vi "Defragment.vi"(11 "Path":path) -> (0 "error out":errorcluster)   [LabVIEW 2019, in "TDMS.lvlib" / "TDMS.lvclass"]
uses:
  TDMS.lvclass
panel:
  in  "Cancel Button":bool
  out "Processing Report Please Wait":dbl(slide) scale=0.0..100.0
  # "%"
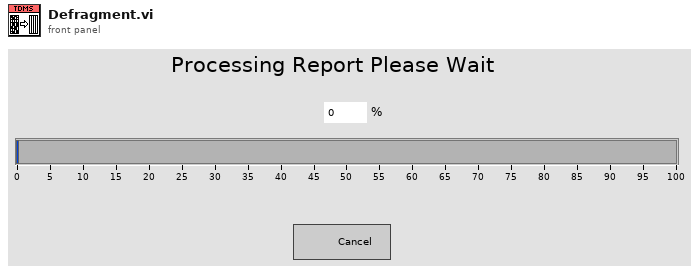
[diagram p1: front panel]
types:
  T1 = enum32{"Invalid", "Standard", "Closed", "Hidden", "Minimized", "Maximized"}
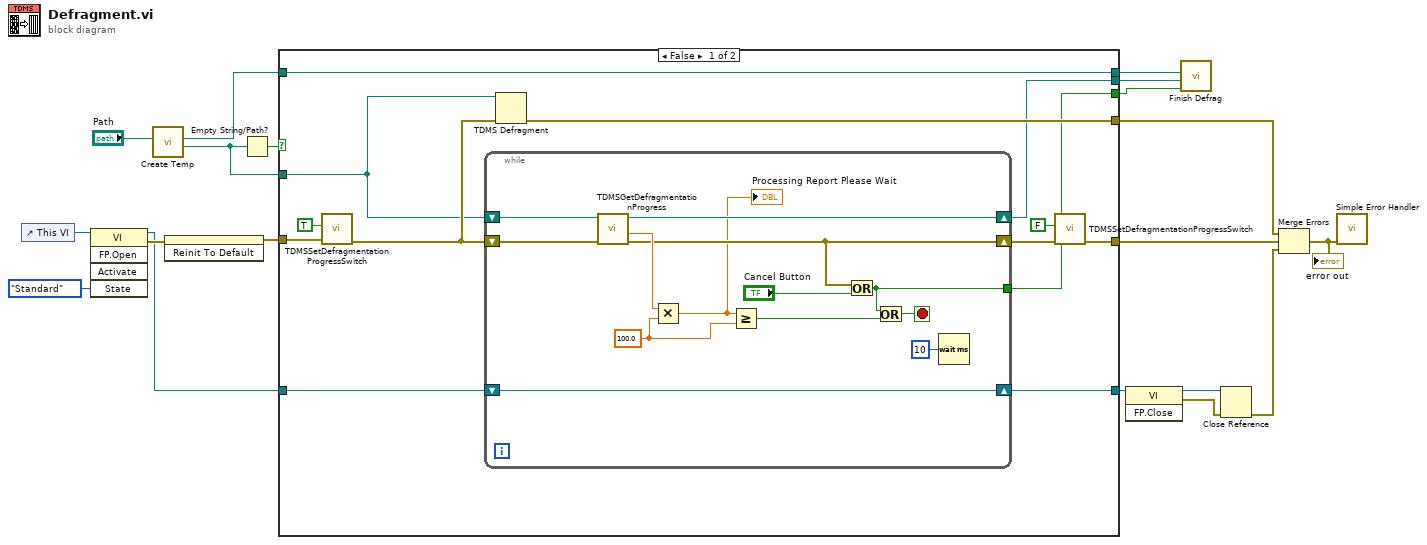
[diagram p0: block diagram]
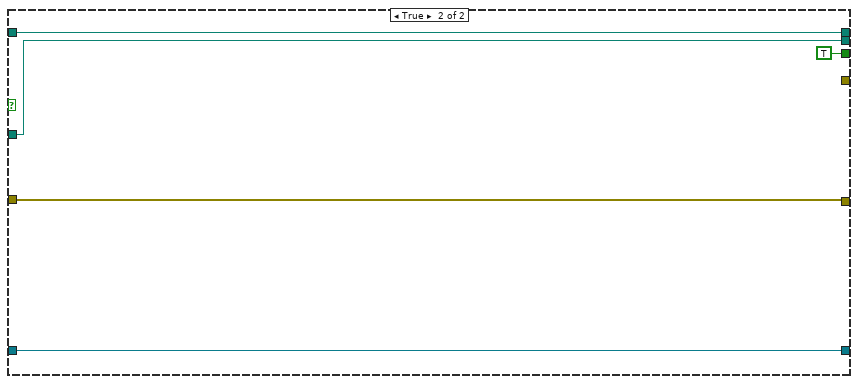
[diagram p2: hidden frame]
diagram:
  n1 = control-ref of="This VI"() -> (w15:refnum<vi>)
  n2 = invoke class="VI" method="FP.Open"(reference=w15, "State"=T1."Standard") -> (reference out=w10:refnum<vi>, error out=w16:errorcluster)  [unwired: 3 in, 3 out]
  n3 = call "Create Temp.vi"("Path"="Path") -> ("Temporary"=w5:path, "Original"=w4:path)  [unwired: 9 in]
  n4 = invoke on="Processing Report Please Wait" class="Slide (strict)" method="Reinit To Default"(error in=w16) -> (error out=w17:errorcluster)  [unwired: 2 in, 2 out]
  n5 = Empty String/Path?(string/path=w5) -> (empty?=w7:bool)
  n6 = case shown="False" w7 {
    tunnel: [w28 w49] -> w19
    tunnel: [w27 _] -> w18
    tunnel: w17 -> [w26 w49]
    tunnel: w10 -> [w25 w50]
    tunnel: [w24 w50] -> w9
    tunnel: w5 -> [w23 w48]
    tunnel: w4 -> [w22 w47]
    tunnel: [w22 w47] -> w3
    tunnel: [w21 TRUE] -> w1
    tunnel: [w20 w48] -> w2
    frame False {
      n7 = call <vilib>:"TDMSSetDefragmentationProgressSwitch.vi"("error in (no error)"=w26, "display defragmentation progress"=TRUE) -> ("error out"=w31:errorcluster)  [unwired: 7 in]
      n8 = while {
        shift-right: [w41] -> w29
        shift-left: w31 -> [w44]
        shift-right: [w43] -> w20
        shift-left: w23 -> [w45]
        shift-right: [w40] -> w24
        shift-left: w25 -> [w40]
        tunnel: [w33] -> w21
        stop <- w35 stop-if-true
        w37 = 100.0 ("y")
        n9 = call <vilib>:"TDMSGetDefragmentationProgress.vi"("error in (no error)"=w44, "file path in"=w45) -> ("error out"=w41:errorcluster, "progress"=w42:dbl, "file path out"=w43:path)  [unwired: 5 in]
        n10 = Multiply(x=w42, y=w37) -> (x*y=w38:dbl)
        "Processing Report Please Wait" <- w38
        n11 = Greater Or Equal?(x=w38, y=w37) -> (x >= y?=w34:bool)
        n12 = Or(x=w41, y="Cancel Button") -> (x .or. y?=w33:bool)
        n13 = Or(x=w33, y=w34) -> (x .or. y?=w35:bool)
        n14 = Wait (ms)(milliseconds to wait=u32 10) -> ()  [unwired: 1 out]
      }
      n15 = TDMS Defragment(4:w31, 7:w23) -> (0:w27:errorcluster)
      n16 = call <vilib>:"TDMSSetDefragmentationProgressSwitch.vi"("error in (no error)"=w29, "display defragmentation progress"=FALSE ("displaySwitch")) -> ("error out"=w28:errorcluster)  [unwired: 7 in]
    }
    frame True {
    }
  }
  n17 = invoke class="VI" method="FP.Close"(reference=w9) -> (reference out=w13:refnum<vi>, error out=w12:errorcluster)  [unwired: 2 in, 1 out]
  n18 = call "Finish Defrag.vi"("Cancelled"=w1, "Temp"=w2, "Original"=w3) -> ()  [unwired: 9 in]
  n19 = Close Reference(reference=w13, error in (no error)=w12) -> (error out=w11:errorcluster)
  n20 = Merge Errors(w18, w19, w11) -> (w8:errorcluster)
  "error out" <- w8
  n21 = call <vilib>:"Simple Error Handler.vi"("error in (no error)"=w8) -> ()  [unwired: 4 in, 5 out]
